vi "Get Count.vi"(8 "error in (no error)":errorcluster, 11 "Mock Data Listener In":refnum<class "Mock Data Listener.lvclass">) -> (0 "error out":errorcluster, 2 "Count":i32, 3 "Mock Data Listener Out":refnum<class "Mock Data Listener.lvclass">)   [LabVIEW 2020, in "Mock Data Listener.lvclass"]
uses:
  Mock Data Listener.lvclass
  Mock Data Listener.lvclass/Mock Data Listener.ctl
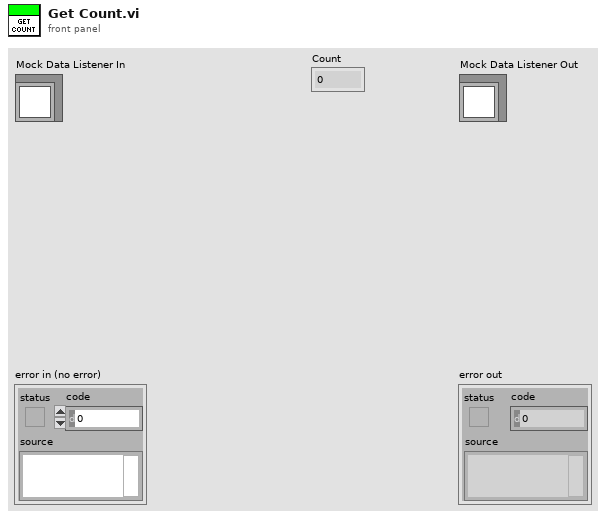
[diagram p1: front panel]
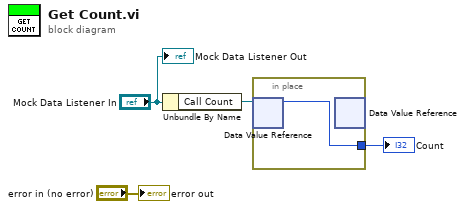
[diagram p0: block diagram]
diagram:
  n1 = Unbundle By Name("Mock Data Listener In") -> ("Call Count"=w2:refnum<data-value>)
  n2 = in-place {
    in-place-border: [w5] -> w1
    n3 = in-place-dvr #1(w2) -> (w5:i32)  [unwired: 1 out]
    n4 = in-place-dvr #1() -> ()  [unwired: 1 in, 2 out]
  }
  "Count" <- w1
  "error out" <- "error in (no error)"
  "Mock Data Listener Out" <- "Mock Data Listener In"
